vi "week9-2.vi"() -> ()   [LabVIEW 2014]
panel:
  in  "stop":bool
  out "State":T1(ring)
  in  "Bound bottom":dbl
  in  "Bound right":dbl
  out "Boolean":bool
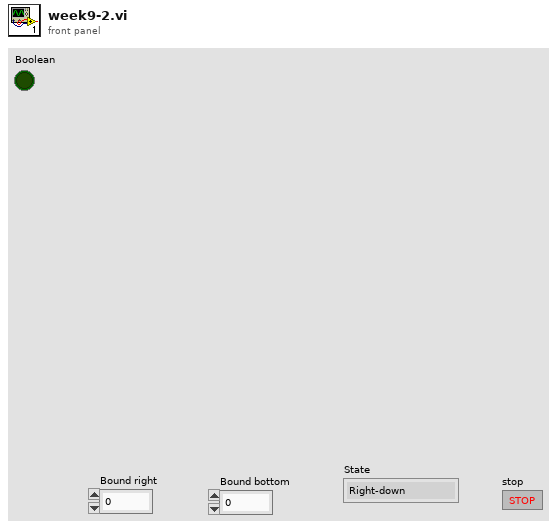
[diagram p1: front panel]
types:
  T1 = enum16{"Right-down", "Right-up", "Left-up", "Left-down"}
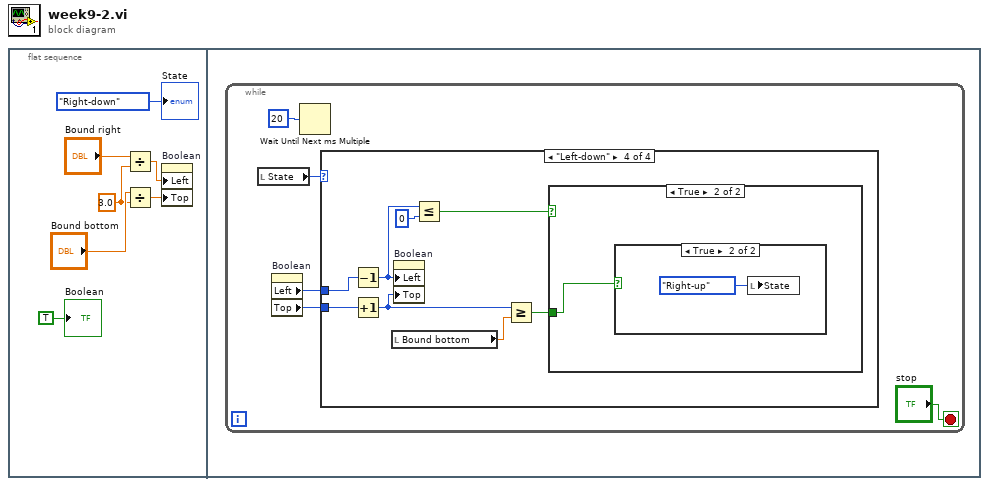
[diagram p0: block diagram]
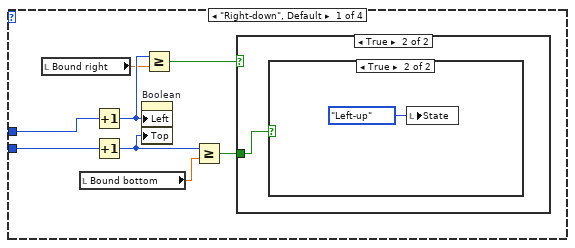
[diagram p2: hidden frame]
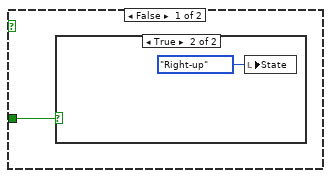
[diagram p3: hidden frame]
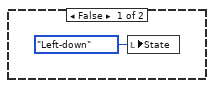
[diagram p5: hidden frame]
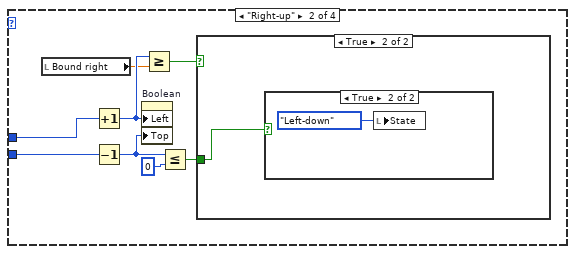
[diagram p6: hidden frame]
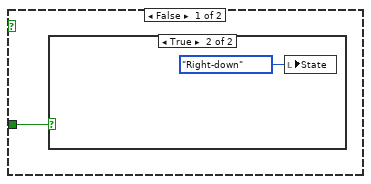
[diagram p7: hidden frame]
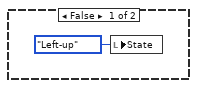
[diagram p9: hidden frame]
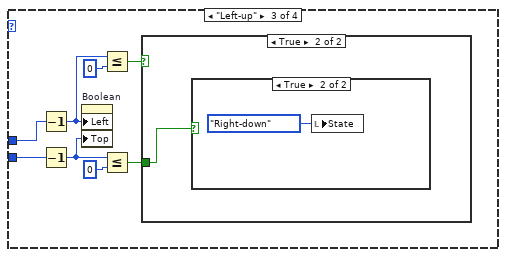
[diagram p10: hidden frame]
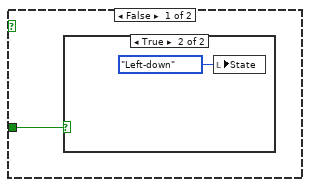
[diagram p11: hidden frame]
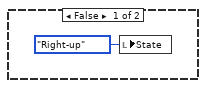
[diagram p13: hidden frame]
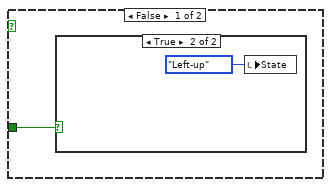
[diagram p14: hidden frame]
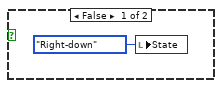
[diagram p16: hidden frame]
diagram:
  n1 = flat-sequence {
    frame #0 {
      w4 = 3.0 ("y")
      n2 = Divide(x="Bound right", y=w4) -> (x/y=w3:dbl)
      n3 = Divide(x="Bound bottom", y=w4) -> (x/y=w2:dbl)
      n4 = property on="Boolean" class="Bool (strict)"("Left"=w3, "Top"=w2) -> ()  [unwired: 2 in, 2 out]
      "Boolean" <- TRUE ("Boolean")
      "State" <- T1."Right-down"
    }
    frame #1 {
      n5 = while {
        stop <- "stop" stop-if-true
        n6 = local read "State"() -> (w10:T1)
        n7 = property on="Boolean" class="Bool (strict)"() -> ("Left"=w8:i32, "Top"=w9:i32)  [unwired: 2 in, 2 out]
        n8 = Wait Until Next ms Multiple(millisecond multiple=u32 20) -> ()  [unwired: 1 out]
        n9 = case shown="\"Left-down\"" w10 {
          tunnel: w8 -> [w20 w28 w41 w54]
          tunnel: w9 -> [w19 w27 w42 w53]
          frame "Right-down", Default {
            n10 = local read "Bound right"() -> (w17:dbl)
            n11 = local read "Bound bottom"() -> (w16:dbl)
            n12 = Increment(x=w20) -> (x+1=w18:i32)
            n13 = Increment(x=w19) -> (x+1=w13:i32)
            n14 = property on="Boolean" class="Bool (strict)"("Left"=w18, "Top"=w13) -> ()  [unwired: 2 in, 2 out]
            n15 = Greater Or Equal?(x=w18, y=w17) -> (x >= y?=w15:bool)
            n16 = Greater Or Equal?(x=w13, y=w16) -> (x >= y?=w14:bool)
            n17 = case shown="True" w15 {
              tunnel: w14 -> [w21 w23]
              frame False {
                n18 = case shown="True" w21 {
                  frame False {
                  }
                  frame True {
                    n19 = local write "State"(T1."Right-up" ("State")) -> ()
                  }
                }
              }
              frame True {
                n20 = case shown="True" w23 {
                  frame False {
                    n21 = local write "State"(T1."Left-down" ("State")) -> ()
                  }
                  frame True {
                    n22 = local write "State"(T1."Left-up" ("State")) -> ()
                  }
                }
              }
            }
          }
          frame "Right-up" {
            n23 = local read "Bound right"() -> (w32:dbl)
            n24 = Increment(x=w28) -> (x+1=w33:i32)
            n25 = Decrement(x=w27) -> (x-1=w29:i32)
            n26 = property on="Boolean" class="Bool (strict)"("Left"=w33, "Top"=w29) -> ()  [unwired: 2 in, 2 out]
            n27 = Greater Or Equal?(x=w33, y=w32) -> (x >= y?=w31:bool)
            n28 = Less Or Equal?(x=w29, y=0) -> (x <= y?=w30:bool)
            n29 = case shown="True" w31 {
              tunnel: w30 -> [w34 w36]
              frame False {
                n30 = case shown="True" w34 {
                  frame False {
                  }
                  frame True {
                    n31 = local write "State"(T1."Right-down" ("State")) -> ()
                  }
                }
              }
              frame True {
                n32 = case shown="True" w36 {
                  frame False {
                    n33 = local write "State"(T1."Left-up" ("State")) -> ()
                  }
                  frame True {
                    n34 = local write "State"(T1."Left-down" ("State")) -> ()
                  }
                }
              }
            }
          }
          frame "Left-up" {
            n35 = Decrement(x=w41) -> (x-1=w46:i32)
            n36 = Decrement(x=w42) -> (x-1=w43:i32)
            n37 = property on="Boolean" class="Bool (strict)"("Left"=w46, "Top"=w43) -> ()  [unwired: 2 in, 2 out]
            n38 = Less Or Equal?(x=w46, y=0) -> (x <= y?=w45:bool)
            n39 = Less Or Equal?(x=w43, y=0) -> (x <= y?=w44:bool)
            n40 = case shown="True" w45 {
              tunnel: w44 -> [w47 w49]
              frame False {
                n41 = case shown="True" w47 {
                  frame False {
                  }
                  frame True {
                    n42 = local write "State"(T1."Left-down" ("State")) -> ()
                  }
                }
              }
              frame True {
                n43 = case shown="True" w49 {
                  frame False {
                    n44 = local write "State"(T1."Right-up" ("State")) -> ()
                  }
                  frame True {
                    n45 = local write "State"(T1."Right-down" ("State")) -> ()
                  }
                }
              }
            }
          }
          frame "Left-down" {
            n46 = Decrement(x=w54) -> (x-1=w59:i32)
            n47 = Increment(x=w53) -> (x+1=w55:i32)
            n48 = local read "Bound bottom"() -> (w58:dbl)
            n49 = property on="Boolean" class="Bool (strict)"("Left"=w59, "Top"=w55) -> ()  [unwired: 2 in, 2 out]
            n50 = Less Or Equal?(x=w59, y=0) -> (x <= y?=w57:bool)
            n51 = Greater Or Equal?(x=w55, y=w58) -> (x >= y?=w56:bool)
            n52 = case shown="True" w57 {
              tunnel: w56 -> [w60 w62]
              frame False {
                n53 = case shown="True" w60 {
                  frame False {
                  }
                  frame True {
                    n54 = local write "State"(T1."Left-up" ("State")) -> ()
                  }
                }
              }
              frame True {
                n55 = case shown="True" w62 {
                  frame False {
                    n56 = local write "State"(T1."Right-down" ("State")) -> ()
                  }
                  frame True {
                    n57 = local write "State"(T1."Right-up" ("State")) -> ()
                  }
                }
              }
            }
          }
        }
      }
    }
  }
